vi "IPC-Modbus-Transfer-EncodeResponse-ModbusTCPFrame.vi"(10 "Modbus TCP Frame Body":string, 11 "MBAP":T1) -> (3 "输出字符串":string)   [LabVIEW 2014]
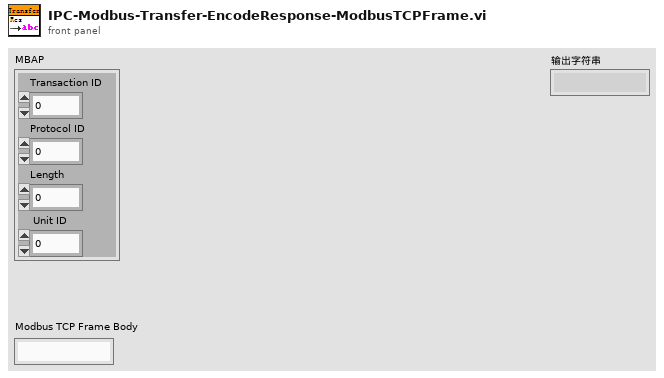
[diagram p1: front panel]
types:
  T1 = cluster{"Transaction ID":u16, "Protocol ID":u16, "Length":u16, " Unit ID":u8}
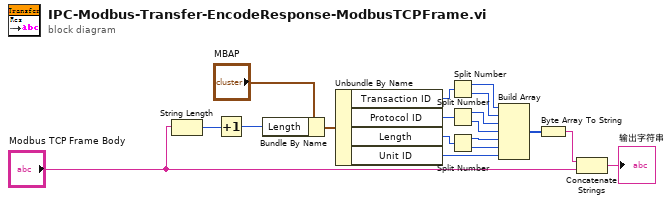
[diagram p0: block diagram]
diagram:
  n1 = String Length(string="Modbus TCP Frame Body") -> (length=w17:i32)
  n2 = Increment(x=w17) -> (x+1=w16:i32)
  n3 = Bundle By Name(cluster="MBAP", "Length"=w16) -> (w14:T1)
  n4 = Unbundle By Name(w14) -> ("Transaction ID"=w13:u16, "Protocol ID"=w10:u16, "Length"=w7:u16, "Unit ID"=w4:u8)
  n5 = Split Number(x=w13) -> (hi(x)=w12:u8, lo(x)=w11:u8)
  n6 = Split Number(x=w10) -> (hi(x)=w9:u8, lo(x)=w8:u8)
  n7 = Split Number(x=w7) -> (hi(x)=w6:u8, lo(x)=w5:u8)
  n8 = Build Array(w12, w11, w9, w8, w6, w5, w4) -> (w3:u8[])
  n9 = Byte Array To String(unsigned byte array=w3) -> (string=w2:string)
  n10 = Concatenate Strings(w2, "Modbus TCP Frame Body") -> (→"输出字符串":string)
